vi "practica2.vi"() -> ()   [LabVIEW 2016]
uses:
  <vilib>/DAQmx/configure/timing.llb/DAQmx Timing (Sample Clock).vi
  <vilib>/DAQmx/create/channels.llb/DAQmx Create Channel (AI-Voltage-Basic).vi
  <vilib>/DAQmx/read.llb/DAQmx Read (Analog 1D DBL NChan 1Samp).vi
  <vilib>/DAQmx/create/channels.llb/DAQmx Create Channel (AO-Voltage-Basic).vi
  <vilib>/DAQmx/write.llb/DAQmx Write (Analog 1D Wfm NChan NSamp).vi
panel:
  in  "Stop Button 2":bool
  out "data":dbl[](array[numeric]) format="%0.2f"
  in  "Stop Button":bool
  out "XY Graph":cluster{dbl[], dbl[]}(graph)
  in  "L 3":dbl(slide) scale=0.0..3.0
  in  "L 2":dbl(slide) scale=0.0..3.0
  in  "L 1":dbl(slide) scale=0.0..3.0
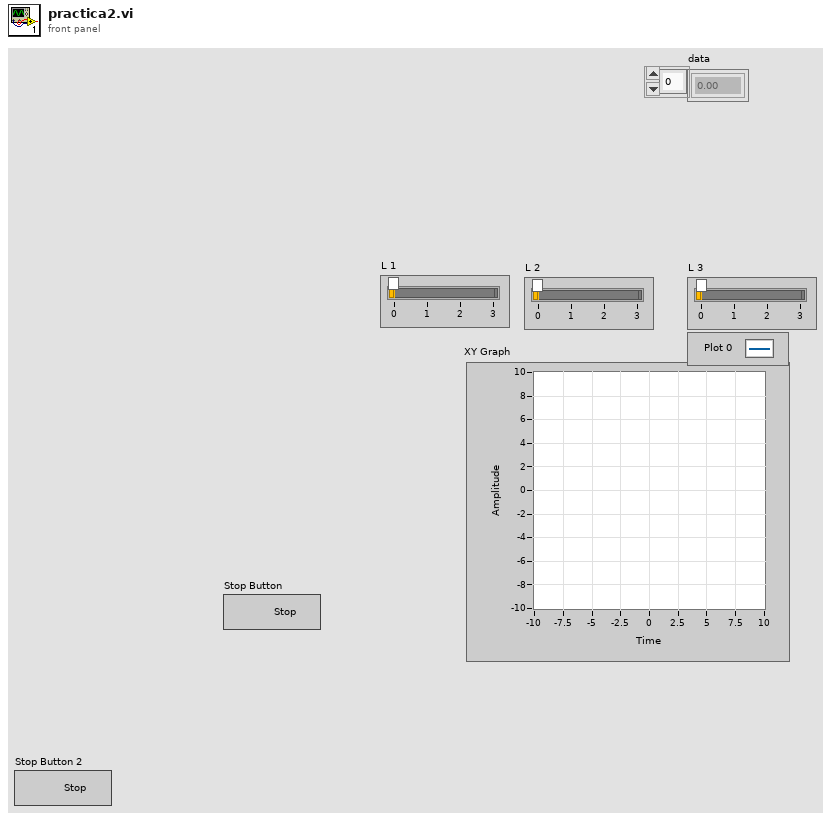
[diagram p1: front panel]
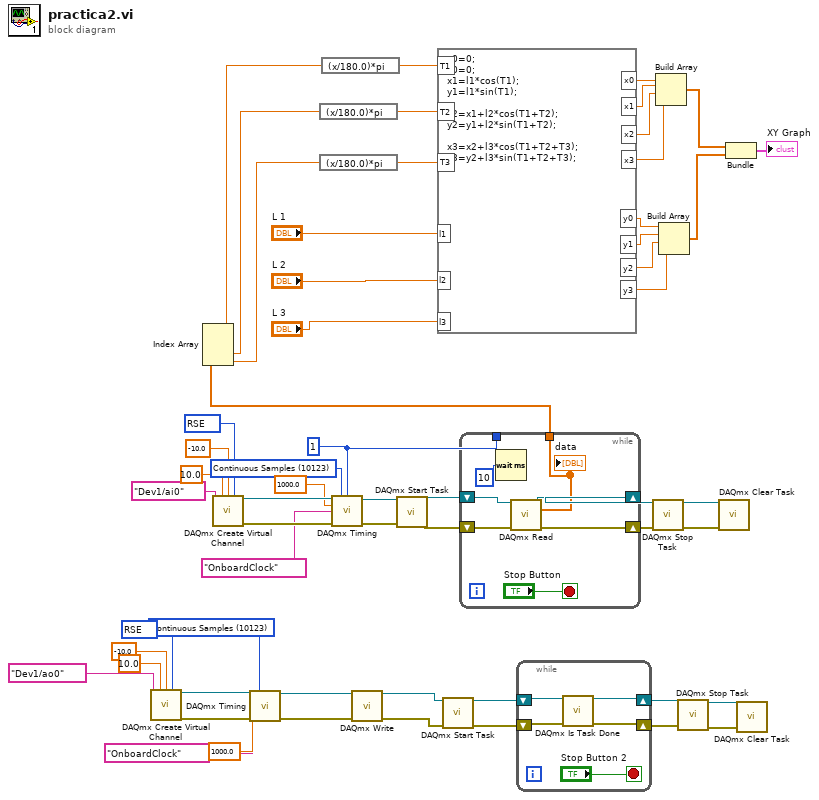
[diagram p0: block diagram]
diagram:
  w14 = 10123 items=["Finite Samples"=10178, "Continuous Samples"=10123, "Hardware Timed Single Point"=12522] ("sample mode")
  w17 = 10083 items=["Default"=-1, "RSE"=10083, "Differential"=10106, "Pseudodifferential"=12529] ("output terminal configuration")
  w29 = 1 ("samples per channel")
  w36 = 10123 items=["Finite Samples"=10178, "Continuous Samples"=10123, "Hardware Timed Single Point"=12522] ("sample mode")
  w39 = 10083 items=["Default"=-1, "RSE"=10083, "NRSE"=10078, "Differential"=10106, "Pseudodifferential"=12529] ("input terminal configuration")
  n1 = call-poly <vilib>:"DAQmx Create Virtual Channel.vi"("maximum value"=10.0, "minimum value"=-10.0, "output terminal configuration"=w17, "physical channels"=tag "Dev1/ao0") -> ("task out"=w16:refnum<k21>, "error out"=w15:errorcluster)  [unwired: 10 in]
  n2 = call-poly <vilib>:"DAQmx Create Virtual Channel.vi"("maximum value"=10.0, "minimum value"=-10.0, "input terminal configuration"=w39, "physical channels"=tag "Dev1/ai0") -> ("task out"=w38:refnum<k21>, "error out"=w37:errorcluster)  [unwired: 10 in]
  n3 = call-poly <vilib>:"DAQmx Timing.vi"("task/channels in"=w16, "sample mode"=w14, "rate"=1000.0, "source"=tag "OnboardClock", "error in"=w15) -> ("task out"=w11:refnum<k21>, "error out"=w10:errorcluster)  [unwired: 9 in]
  n4 = call-poly <vilib>:"DAQmx Timing.vi"("task/channels in"=w38, "sample mode"=w36, "samples per channel"=w29, "rate"=1000.0, "source"=tag "OnboardClock", "error in"=w37) -> ("task out"=w33:refnum<k21>, "error out"=w32:errorcluster)  [unwired: 8 in]
  n5 = call-poly <vilib>:"DAQmx Write.vi"("task/channels in"=w11, "error in"=w10) -> ("task out"=w9:refnum<k21>, "error out"=w8:errorcluster)  [unwired: 11 in, 1 out]
  n6 = call <vilib>:"DAQmx Start Task.vi"("task/channels in"=w33, "error in"=w32) -> ("task out"=w31:refnum<k21>, "error out"=w30:errorcluster)  [unwired: 12 in]
  n7 = call <vilib>:"DAQmx Start Task.vi"("task/channels in"=w9, "error in"=w8) -> ("task out"=w7:refnum<k21>, "error out"=w6:errorcluster)  [unwired: 12 in]
  n8 = while {
    tunnel: w29 -> [_]
    shift-right: [w63] -> w28
    shift-left: w31 -> [w65]
    shift-right: [w62] -> w27
    shift-left: w30 -> [w64]
    tunnel: [w59] -> w24
    stop <- "Stop Button" stop-if-true
    n9 = Wait (ms)(milliseconds to wait=u32 10) -> ()  [unwired: 1 out]
    n10 = call-poly <vilib>:"DAQmx Read.vi"("task/channels in"=w65, "error in"=w64) -> ("task out"=w63:refnum<k21>, "data"=w59:dbl[], "error out"=w62:errorcluster)  [unwired: 11 in]
    "data" <- w59
  }
  n11 = Index Array(array=w24) -> (element #1=w21:dbl, element #2=w22:dbl, element #3=w23:dbl)  [unwired: 3 in]
  n12 = expression code="(x/180.0)*pi" ("degrees to radians")(w22) -> (w56:dbl)
  n13 = expression code="(x/180.0)*pi" ("degrees to radians")(w23) -> (w49:dbl)
  n14 = expression code="(x/180.0)*pi" ("degrees to radians")(w21) -> (w57:dbl)
  n15 = formula code="x0=0;\ny0=0;\nx1=l1*cos(T1);\ny1=l1*sin(T1);\n\nx2=x1+l2*cos(T1+T2);\ny2=y1+l2*sin(T1+T2);\n\nx3=x2+l3*cos(T1+T2+T3);\ny3=y2+l3*sin(T1+T2+T3);"("T1"=w57, "l1"="L 1", "T2"=w56, "T3"=w49, "l2"="L 2", "l3"="L 3") -> ("x0"=w55:dbl, "x1"=w54:dbl, "y0"=w53:dbl, "y1"=w52:dbl, "x2"=w48:dbl, "y2"=w47:dbl, "y3"=w44:dbl, "x3"=w43:dbl)
  n16 = while {
    shift-right: [w67] -> w5
    shift-left: w7 -> [w69]
    shift-right: [w66] -> w4
    shift-left: w6 -> [w68]
    stop <- "Stop Button 2" stop-if-true
    n17 = call <vilib>:"DAQmx Is Task Done.vi"("task/channels in"=w69, "error in"=w68) -> ("task out"=w67:refnum<k21>, "error out"=w66:errorcluster)  [unwired: 11 in, 1 out]
  }
  n18 = call <vilib>:"DAQmx Stop Task.vi"("task/channels in"=w28, "error in"=w27) -> ("task out"=w26:refnum<k21>, "error out"=w25:errorcluster)  [unwired: 12 in]
  n19 = Build Array(w55, w54, w48, w43) -> (w51:dbl[])
  n20 = Build Array(w53, w52, w47, w44) -> (w50:dbl[])
  n21 = call <vilib>:"DAQmx Stop Task.vi"("task/channels in"=w5, "error in"=w4) -> ("task out"=w3:refnum<k21>, "error out"=w2:errorcluster)  [unwired: 12 in]
  n22 = call <vilib>:"DAQmx Clear Task.vi"("task in"=w26, "error in"=w25) -> ()  [unwired: 13 in, 1 out]
  n23 = Bundle(w51, w50) -> (→"XY Graph":cluster{dbl[], dbl[]})  [unwired: 1 in]
  n24 = call <vilib>:"DAQmx Clear Task.vi"("task in"=w3, "error in"=w2) -> ()  [unwired: 13 in, 1 out]
